vi "3_AdvancedDemo_TH260T3.vi"() -> ()   [LabVIEW 2017]
uses:
  Types/TH260_InputChannel.ctl
  Types/TH260_UIThread_Cmds.ctl
  Types/TH260_UIThread_Data.ctl
  _lib/PQ/TimeHarp260/TH260_InitInfo.ctl
  Types/TH260_DataProcThread_QData.ctl
  Types/TH260_DataProcThread_QCmds.ctl
  Types/TH260_VisThread_QData.ctl
  Types/TH260_VisThread_QCmds.ctl
  Types/TH260_VisThread_Data.ctl
  _lib/PQ/TimeHarp260/TH260_MeasMode.ctl
  _lib/PQ/TimeHarp260/TH260_TimingMode.ctl
  <vilib>/Utility/error.llb/DialogType.ctl
  _lib/PQ/TimeHarp260/th260lib_x86_x64_UIThread.llb/TH260_DllPath_global.vi
  <vilib>/Utility/error.llb/Error Cluster From Error Code.vi
  _lib/PQ/TimeHarp260/TH260_LibVersion_global.vi
  <vilib>/ErrorRing/Error Ring.xnode
panel:
  in  "Settings":bool=TRUE
  in  "Run continuously":bool caption="Conti."
  in  "Start":bool
  in  "Scale":bool
  out "CountRates":i32[](graph)
  in  "HistoAcqTime":dbl=1.0 caption="Int.Time    s" min=0.1 max=360000.0 step=0.1
  in  "AcqTime":i32=360000000 caption="T3Acq.   ms" min=1 max=360000 step=1
  in  "Binning":i32(ring) caption="Resol.      ps" items=["250", "500", "1000", "2000", "4000", "8000", "16000", "32000", "64000", "128000", "256000", "512000", "1024000", "2048000", "4096000", "8192000", "16384000", "32768000", "65536000", "131072000", "262144000", "524288000"]
  in  "HistoOffset":i32 caption="Offset      ns" min=0 max=500000 step=1
  out "DeltaT":dbl=inf caption="Resol.     ms" format="%.2f"
  in  "BitShift":i32=15 min=0 max=32 step=1
  in  "OvlLevel":u32=65536 caption="Ovl.Level" min=1024 max=65536 step=1024
  in  "StopOvl.":bool=TRUE
  out "TTraceGraph":T1(graph)
  out "HistoGraph":cluster{dbl, "Resol":dbl, "Histos":u32[][]}(graph)
  in  "SyncTrgEdge":i32(ring) caption="Edge" items=["falling", "rising"]
  in  "SyncTrgLevel":i32=-100 caption="Level        mV" min=-1200 max=1200 step=1
  in  "SyncCFDLevel":i32=-100 caption="Level        mV" min=-1200 max=0 step=1
  in  "SyncZeroX":i32=-10 caption="ZeroCr.    mV" min=-40 max=0 step=1
  in  "SyncDivider":i32(ring)=3 caption="Divider" items=["1", "2", "4", "8"]
  in  "SyncOffset":i32 caption="Offset        ps" min=-99999 max=99999 step=1
  in  "Channels":T2[](array[typedef])=[{"Name"="Inp.Chan 1", "Enable"=TRUE, "Offset"=0, "CFDLevel"=50, "ZeroX"=10, "dtcode"=0, "TrgLevel"=-100, "TrgEdge"=0}, {"Name"="Inp.Chan 2", "Enable"=TRUE, "Offset"=0, "CFDLevel"=50, "ZeroX"=10, "dtcode"=0, "TrgLevel"=-100, "TrgEdge"=0}, {"Name"="Inp.Chan 3", "Enable"=TRUE, "Offset"=0, "CFDLevel"=50, "ZeroX"=10, "dtcode"=0, "TrgLevel"=-100, "TrgEdge"=0}, {"Name"="Inp.Chan 4", "Enable"=TRUE, "Offset"=0, "CFDLevel"=50, "ZeroX"=10, "dtcode"=0, "TrgLevel"=-100, "TrgEdge"=0}, {"Name"="Inp.Chan 5", "Enable"=TRUE, "Offset"=0, "CFDLevel"=50, "ZeroX"=10, "dtcode"=0, "TrgLevel"=-100, "TrgEdge"=0}, {"Name"="Inp.Chan 6", "Enable"=TRUE, "Offset"=0, "CFDLevel"=50, "ZeroX"=10, "dtcode"=0, "TrgLevel"=-100, "TrgEdge"=0}, {"Name"="Inp.Chan 7", "Enable"=TRUE, "Offset"=0, "CFDLevel"=50, "ZeroX"=10, "dtcode"=0, "TrgLevel"=-100, "TrgEdge"=0}, {"Name"="Inp.Chan 8", "Enable"=TRUE, "Offset"=0, "CFDLevel"=50, "ZeroX"=10, "dtcode"=0, "TrgLevel"=-100, "TrgEdge"=0}] {"TrgEdge" items=["falling", "rising"]; "TrgLevel" min=-1200 max=1200 step=1; "dtcode" items=["24", "44", "66", "88", "112", "135", "160", "180"]; "ZeroX" min=-40 max=0 step=1; "Offset" min=-99999 max=99999 step=1; "CFDLevel" min=-1200 max=0 step=1}
  out "SyncRate":string="Sync Rate: 0 cps\n"
  out "OverRun":bool caption="Overrun:"
  out "Status":string="Elements in Q: 0"
  # "Histogram"
  # "Time Trace"
  # "Sync"
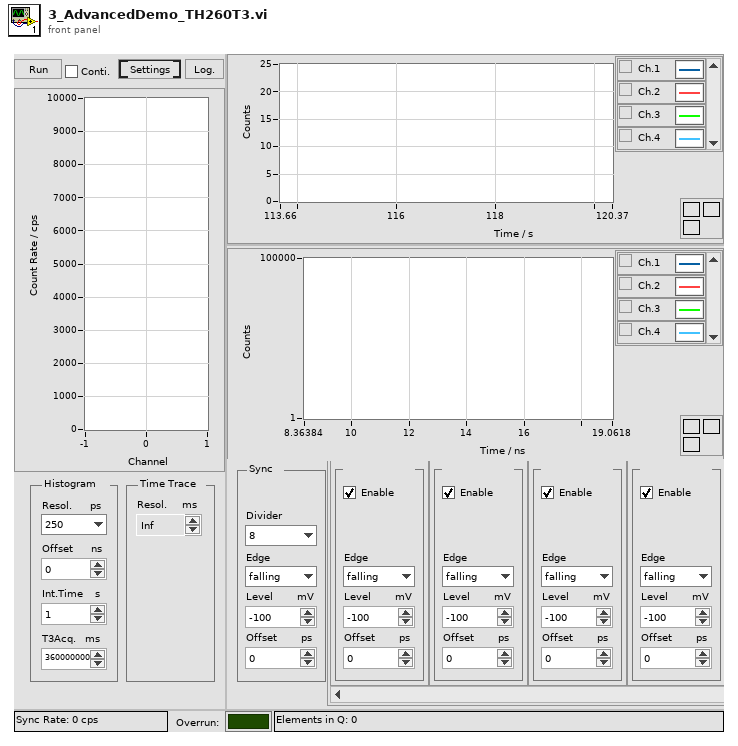
[diagram p1: front panel]
types:
  T1 = cluster{dbl, "Resolution":dbl, "Histogram":u32[][]}
  T2 = typedef "TH260_InputChannel.ctl" = cluster{"Name":string, "Enable":bool, "Offset":i32, "CFDLevel":i32, "ZeroX":i32, "dtcode":i32, "TrgLevel":i32, "TrgEdge":i32}
  T3 = typedef "TH260_DataProcThread_QCmds.ctl" = enum16{"Exit", "Proc", "Init", "SetShift", "SetNumChannels", "SetHistAcqTime"}
  T4 = typedef "TH260_VisThread_Data.ctl" = cluster{"Resol":dbl, "DeltaT":dbl, "NumChannels":i32}
  T5 = typedef "TH260_VisThread_QData.ctl" = cluster{"Histos":u32[][], "Cmd":T6, "TimeTrace":u32[][], "Bin":i32, "Total bin":u64, "Status":string, "Resol":dbl, "DeltaT":dbl, "nChannels":i32}
  T6 = typedef "TH260_VisThread_QCmds.ctl" = enum16{"_none_", "Resol", "nChannels", "DeltaT", "Histo", "TTrace", "Status"}
  T7 = typedef "TH260_DataProcThread_QData.ctl" = cluster{"Cmd":T3, "nActual":i32, "Buffer":u32[], "TickCount":u32, "Param":i32}
  T8 = typedef "TH260_UIThread_Data.ctl" = cluster{"Init Info":T9, "DevIdx":i32, "Channels":T2[], "CurrentChannels":i32[], "AcqTime":i32, "Binning":i32, "HistoOffset":i32, "HistoLen":i32, "StopOvl.":bool, "OvlLevel":u32, "StartMeas":bool, "HistoLength":i32, "Resolution":dbl, "Run cont.":bool, "Status":string, "SyncRate":i32, "BitShift":i32, "HistoAcqTime":dbl, "SyncTrgEdge":i32, "SyncTrgLevel":i32, "SyncCFDLevel":i32, "SyncZeroX":i32, "SyncDivider":i32, "SyncOffset":i32}
  T9 = typedef "TH260_InitInfo.ctl" = cluster{"Library Version":string, "Serial No.":string, "Model":string, "Partnum":string, "Version":string, "features":i32, "nchannels":i32, "Base Resolution":dbl, "Bin Steps":i32}
  T10 = typedef "TH260_UIThread_Cmds.ctl" = enum16{"Idle", "Init", "SetInpChanEnable", "SetInpChanOffset", "SetInpChanCFD", "SetInpChanTrg", "SetInpChanDeadtime", "SetSyncDivider", "SetSyncCFD", "SetSyncTrg", "SetSyncOffset", "SetBinning", "SetHistoOffset", "SetHistoLen", "SetStopOvl", "SetBitShift", "SetHistoAcqTime", "GetRates", "StartMeas", "StopMeas", "AbortMeas", "GetResolution", "GetHisto", "ReadFiFo", "WriteStatus", "Resize", "EnableControls", "DisableControls", "Error", "Exit"}
  T11 = enum8{"Enabled", "Disabled", "Disabled and Grayed Out"}
  T12 = typedef "TH260_TimingMode.ctl" = i32
  T13 = typedef "TH260_MeasMode.ctl" = i32
  T14 = typedef "DialogType.ctl" = u16
  T15 = cluster{"T0":dbl, "dt":dbl, "TimeTrace_out":u32[][]}
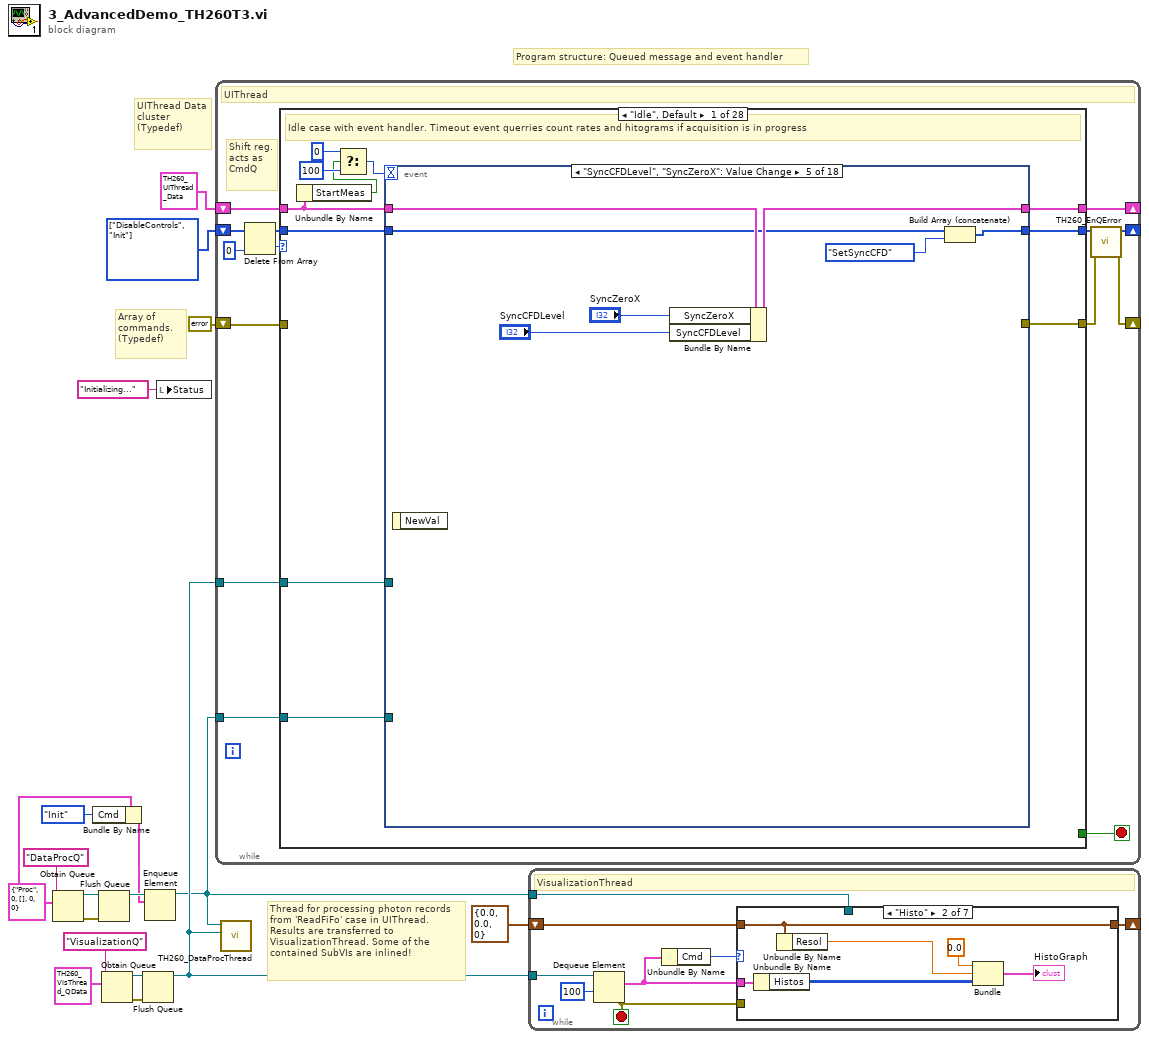
[diagram p0: block diagram]
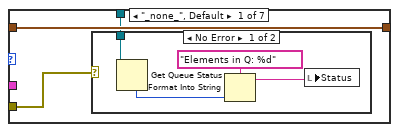
[diagram p2: hidden frame]
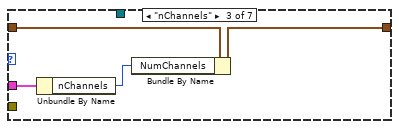
[diagram p4: hidden frame]
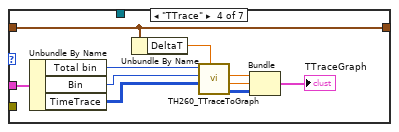
[diagram p5: hidden frame]
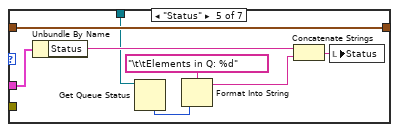
[diagram p6: hidden frame]
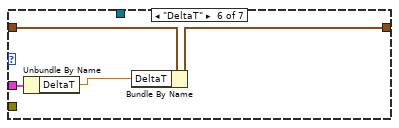
[diagram p7: hidden frame]
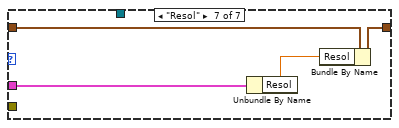
[diagram p8: hidden frame]
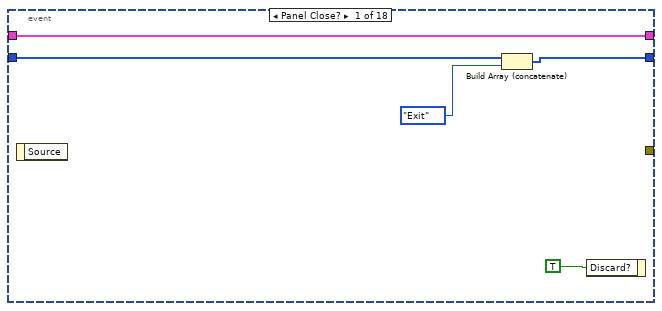
[diagram p9: hidden frame]
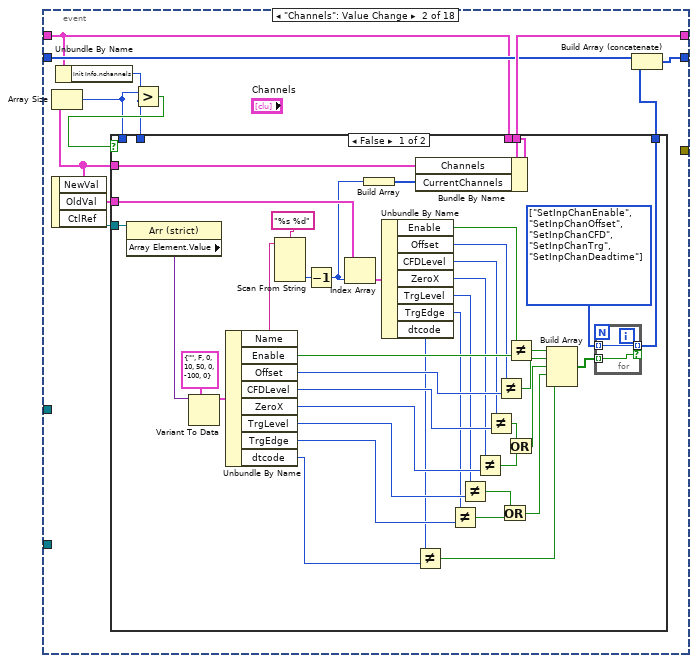
[diagram p10: hidden frame]
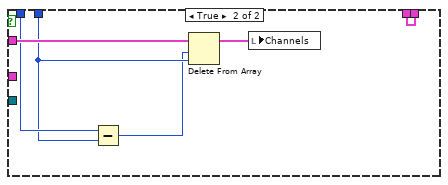
[diagram p11: hidden frame]
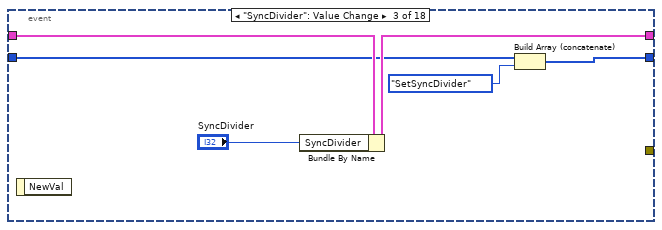
[diagram p12: hidden frame]
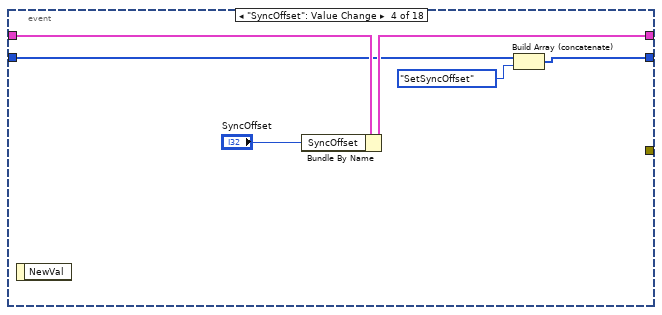
[diagram p13: hidden frame]
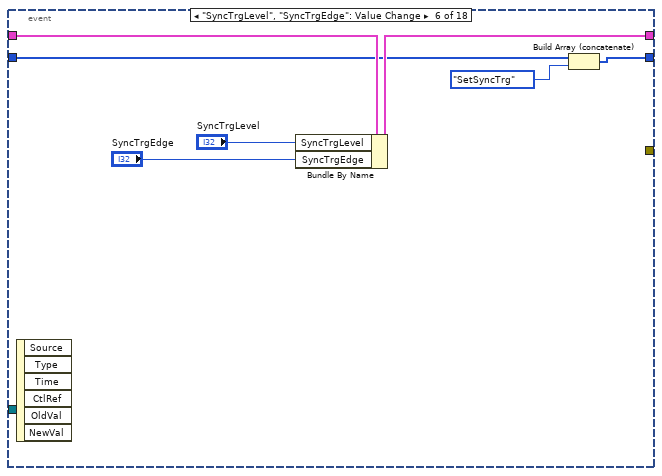
[diagram p14: hidden frame]
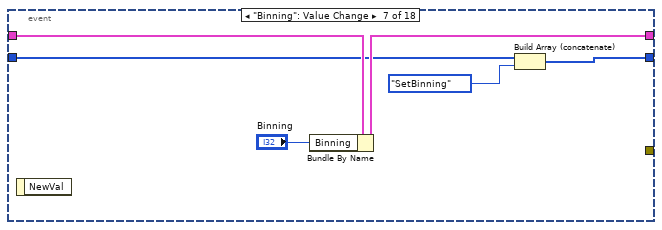
[diagram p15: hidden frame]
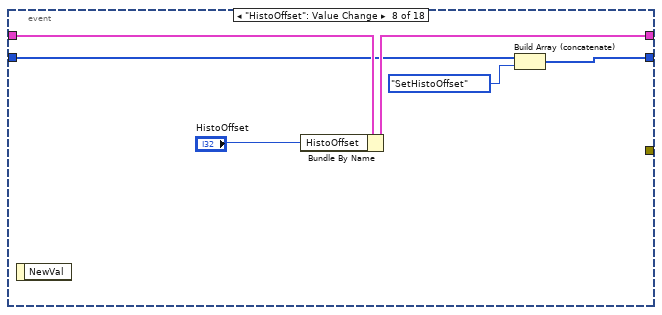
[diagram p16: hidden frame]
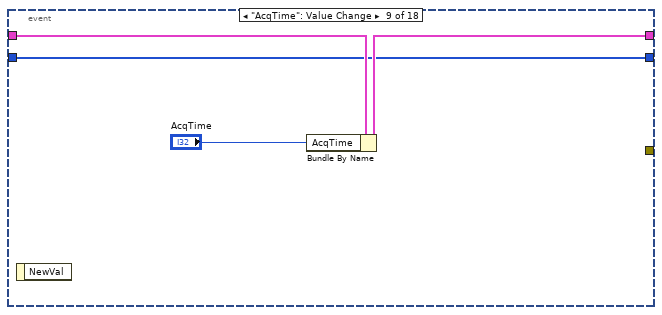
[diagram p17: hidden frame]
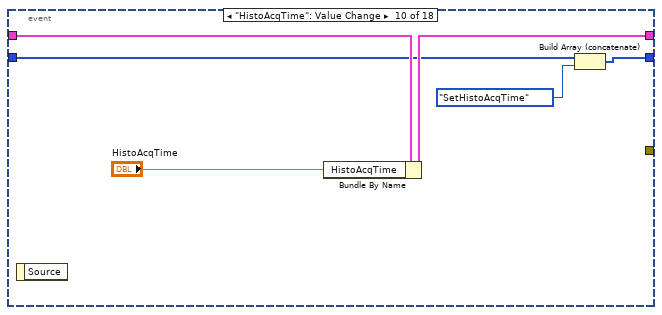
[diagram p18: hidden frame]
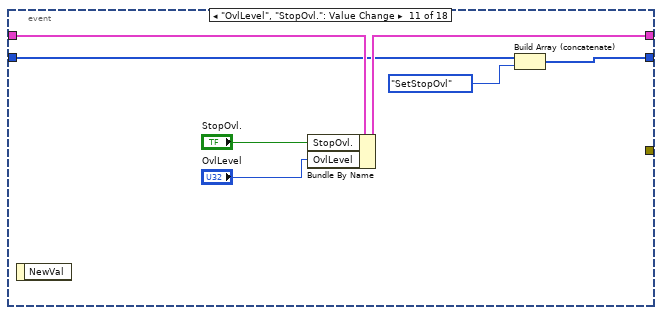
[diagram p19: hidden frame]
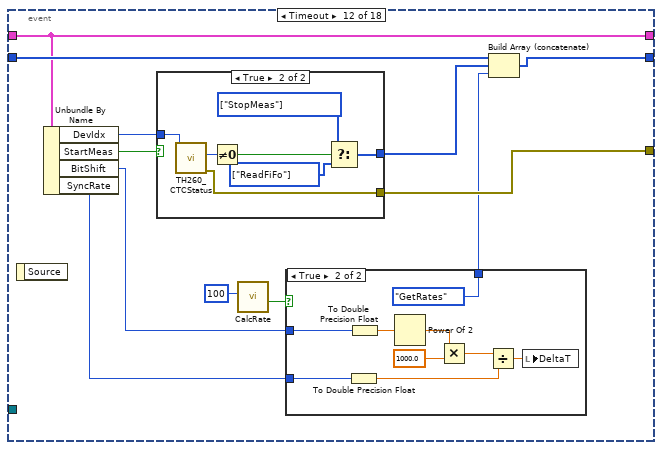
[diagram p20: hidden frame]
diagram:
  w4 = T7 {"Cmd"=enum."Proc", "nActual"=0, "Buffer"=[], "TickCount"=0, "Param"=0} ("MH_DataProcThread_QData")
  w17 = T10[] [enum."DisableControls", enum."Init"] items=["Idle", "Init", "SetInpChanEnable", "SetInpChanOffset", "SetInpChanCFD", "SetInpChanTrg", "SetInpChanDeadtime", "SetSyncDivider", "SetSyncCFD", "SetSyncTrg", "SetSyncOffset", "SetBinning", "SetHistoOffset", "SetHistoLen", "SetStopOvl", "SetBitShift", "SetHistoAcqTime", "GetRates", "StartMeas", "StopMeas", "AbortMeas", "GetResolution", "GetHisto", "ReadFiFo", "WriteStatus", "Resize", "EnableControls", "DisableControls", "Error", "Exit"]
  # "Thread for processing photon records from 'ReadFiFo' case in UIThread. Results are transferred to VisualizationThread. Some of the contained SubVIs are inlined!"
  # "Array of commands.\n(Typedef)"
  # "Program structure: Queued message and event handler"
  # "UIThread Data cluster\n(Typedef)"
  n1 = Obtain Queue(name (unnamed)="DataProcQ", element data type=w4) -> (queue out=w14:refnum<queue>, error out=w13:errorcluster)  [unwired: 3 in, 1 out]
  n2 = Bundle By Name(cluster=w4, "Cmd"=TH260_DataProcThread_QCmds."Init") -> (w2:T7)
  n3 = Flush Queue(queue=w14, error in (no error)=w13) -> (queue out=w5:refnum<queue>)  [unwired: 2 out]
  n4 = Obtain Queue(name (unnamed)="VisualizationQ", element data type=T5 {"Histos"=[], "Cmd"=enum."_none_", "TimeTrace"=[], "Bin"=0, "Total bin"=0, "Status"="", "Resol"=0.0, "DeltaT"=0.0, "nChannels"=0} ("MH_GUIThread_QData")) -> (queue out=w12:refnum<queue>, error out=w11:errorcluster)  [unwired: 3 in, 1 out]
  n5 = Flush Queue(queue=w12, error in (no error)=w11) -> (queue out=w7:refnum<queue>)  [unwired: 2 out]
  n6 = Enqueue Element(queue=w5, element=w2) -> (queue out=w1:refnum<queue>)  [unwired: 2 in, 2 out]
  n7 = local write "Status"("Initializing..." ("Status")) -> ()
  n8 = while {
    shift-right: [w21] -> _
    shift-left: w17 -> [w28]
    shift-right: [w31] -> _
    shift-left: T8 {"Init Info"={"Library Version"="", "Serial No."="", "Model"="", "Partnum"="", "Version"="", "features"=0, "nchannels"=0, "Base Resolution"=0.0, "Bin Steps"=0}, "DevIdx"=0, "Channels"=[], "CurrentChannels"=[], "AcqTime"=1, "Binning"=1, "HistoOffset"=1, "HistoLen"=1024, "StopOvl."=FALSE, "OvlLevel"=1024, "StartMeas"=FALSE, "HistoLength"=0, "Resolution"=0.0, "Run cont."=FALSE, "Status"="", "SyncRate"=0, "BitShift"=0, "HistoAcqTime"=0.0, "SyncTrgEdge"=50, "SyncTrgLevel"=0, "SyncCFDLevel"=-100, "SyncZeroX"=10, "SyncDivider"=1, "SyncOffset"=0} -> [w30]
    shift-right: [w23] -> _
    shift-left: errorcluster {"status"=FALSE, "code"=0, "source"=""} ("error IO") -> [w29]
    tunnel: w1 -> [w20]
    tunnel: w7 -> [w19]
    stop <- w32 stop-if-true
    # "Shift reg.\nacts as\nCmdQ"
    # "UIThread"
    n9 = Delete From Array(array=w28, index=0) -> (deleted portion=w26:T10, array with subset deleted=w25:T10[])  [unwired: 1 in]
    n10 = case shown="\"Idle\", Default" w26 {
      tunnel: [w43 w297 w331 w345 w359 w374 w389 w405 w414 w420 w422 w429 w437 w443 w463 w475 w487 w507 w513 w526 w543 w544 w570 w583 w590 w602 w608 w614] -> w22
      tunnel: [_ _ _ _ _ _ _ _ _ _ _ _ _ _ _ _ _ _ _ _ _ _ _ _ _ _ _ TRUE] -> w32
      tunnel: [w42 w278 w334 w348 w362 w377 w392 w407 w415 w421 w426 w433 w438 w444 w448 w465 w477 w511 w516 w528 w539 w554 w569 w571 w589 w601 w609 w617] -> w31
      tunnel: w30 -> [w39 w283 w334 w348 w362 w377 w392 w407 w415 w421 w426 w433 w438 w444 w448 w465 w478 w511 w517 w529 w540 w554 w569 w571 w589 w601 w609 w617]
      tunnel: [w40 w301 w332 w346 w360 w375 w390 w403 w413 w419 w425 w432 w436 w442 _ _ w486 w510 w519 w531 w541 w549 _ _ _ _ _ w615] -> w24
      tunnel: w29 -> [_ _ _ _ _ _ _ _ _ _ _ _ _ _ _ _ _ _ _ _ _ _ _ _ _ _ w610 _]
      tunnel: w25 -> [w41 w298 w331 w345 w359 w374 w389 w405 w414 w420 w422 w428 w437 w443 w463 w475 w487 w508 w514 w526 w543 w545 w570 w583 w590 w602 _ w614]
      tunnel: w20 -> [w34 w276 _ _ _ _ _ _ _ _ _ _ _ _ w449 w466 _ w504 _ _ _ w546 _ _ _ _ _ w613]
      tunnel: w19 -> [w33 w268 _ _ _ _ _ _ _ _ _ _ _ _ w450 _ _ _ _ _ w536 _ _ _ _ _ _ w612]
      frame "Idle", Default {
        # "Idle case with event handler. Timeout event querries count rates and hitograms if acquisition is in progress"
        n11 = Unbundle By Name(w39) -> ("StartMeas"=w37:bool)
        n12 = Select(t=0, s=w37, f=100) -> (s? t:f=w36:i32)
        n13 = event shown="[4] \"SyncCFDLevel\", \"SyncZeroX\": Value Change" {
          selector: _ -> [_ _ _ _ _ _ _ _ _ _ _ _ _ _ _ _ _ _]
          dyn-events: _ -> [_ _ _ _ _ _ _ _ _ _ _ _ _ _ _ _ _ _]
          timeout: w36 -> [_ _ _ _ _ _ _ _ _ _ _ _ _ _ _ _ _ _]
          tunnel: [w44 w54 w109 w115 w122 w129 w135 w141 w146 w151 w158 w173 w191 w203 w221 w227 w235 w245] -> w43
          tunnel: [w47 w57 w112 w118 w125 w132 w138 w144 w148 w154 w161 w172 w195 w202 w219 w226 w234 w248] -> w42
          tunnel: w39 -> [w47 w53 w113 w119 w126 w133 w139 w145 w149 w155 w162 w172 w196 w200 w220 w226 w234 w248]
          tunnel: w41 -> [w46 w56 w111 w117 w124 w131 w137 w143 w146 w152 w160 w174 w192 w204 w221 w227 w235 w246]
          tunnel: [_ _ _ _ _ _ _ _ _ _ _ w168 _ _ _ _ _ _] -> w40
          tunnel: w34 -> [_ _ _ _ _ _ _ _ _ _ _ _ _ _ _ _ _ _]
          tunnel: w33 -> [_ _ _ _ _ _ _ _ _ _ _ _ _ _ _ _ _ _]
          event Panel Close? {
            n14 = event-data() -> ()  [unwired: 1 in, 1 out]
            n15 = Build Array (concatenate)(w46, TH260_UIThread_Cmds."Exit") -> (w44:T10[])
            n16 = event-data("Discard?"=TRUE) -> ()  [unwired: 1 in, 1 out]
          }
          event "Channels": Value Change {
            n17 = event-data() -> ("NewVal"=w52:T2[], "OldVal"=w58:T2[], "CtlRef"=w59:refnum<vi>)  [unwired: 1 in]
            n18 = Array Size(array=w52) -> (size(s)=w49:i32)
            n19 = Unbundle By Name(w53) -> ("Init Info.nchannels"=w50:i32)
            n20 = Greater?(x=w49, y=w50) -> (0:w51:bool)
            n21 = case shown="False" w51 {
              tunnel: w59 -> [w99 _]
              tunnel: w58 -> [w93 _]
              tunnel: [w76 w107] -> w57
              tunnel: [w74 _] -> w55
              tunnel: w53 -> [w71 w107]
              tunnel: w52 -> [w70 w106]
              tunnel: w50 -> [_ w104]
              tunnel: w49 -> [_ w105]
              frame False {
                w77 = T10[] [enum."SetInpChanEnable", enum."SetInpChanOffset", enum."SetInpChanCFD", enum."SetInpChanTrg", enum."SetInpChanDeadtime"] items=["Idle", "Init", "SetInpChanEnable", "SetInpChanOffset", "SetInpChanCFD", "SetInpChanTrg", "SetInpChanDeadtime", "SetSyncDivider", "SetSyncCFD", "SetSyncTrg", "SetSyncOffset", "SetBinning", "SetHistoOffset", "SetHistoLen", "SetStopOvl", "SetBitShift", "SetHistoAcqTime", "GetRates", "StartMeas", "StopMeas", "AbortMeas", "GetResolution", "GetHisto", "ReadFiFo", "WriteStatus", "Resize", "EnableControls", "DisableControls", "Error", "Exit"]
                n22 = property class="Arr (strict)"(reference=w99) -> ("Array Element.Value"=w98:variant)  [unwired: 1 in, 2 out]
                n23 = Variant To Data(type=T2 {"Name"="", "Enable"=FALSE, "Offset"=0, "CFDLevel"=10, "ZeroX"=50, "dtcode"=0, "TrgLevel"=-100, "TrgEdge"=0} ("Channel"), Variant=w98) -> (data=w75:T2)  [unwired: 1 in, 1 out]
                n24 = Unbundle By Name(w75) -> ("Name"=w96:string, "Enable"=w90:bool, "Offset"=w88:i32, "CFDLevel"=w86:i32, "ZeroX"=w84:i32, "TrgLevel"=w68:i32, "TrgEdge"=w66:i32, "dtcode"=w61:i32)
                n25 = Scan From String(format string="%s %d", input string=w96) -> (output 2=w94:i32)  [unwired: 5 in, 3 out]
                n26 = Decrement(x=w94) -> (x-1=w73:i32)
                n27 = Index Array(array=w93, index=w73) -> (element=w92:T2)
                n28 = Build Array(w73) -> (w72:i32[])
                n29 = Unbundle By Name(w92) -> ("Enable"=w91:bool, "Offset"=w89:i32, "CFDLevel"=w87:i32, "ZeroX"=w85:i32, "TrgLevel"=w69:i32, "TrgEdge"=w67:i32, "dtcode"=w62:i32)
                n30 = Not Equal?(x=w62, y=w61) -> (x != y?=w60:bool)
                n31 = Bundle By Name(cluster=w71, "Channels"=w70, "CurrentChannels"=w72) -> (w76:T8)
                n32 = Not Equal?(x=w67, y=w66) -> (x != y?=w64:bool)
                n33 = Not Equal?(x=w69, y=w68) -> (x != y?=w65:bool)
                n34 = Not Equal?(x=w85, y=w84) -> (x != y?=w79:bool)
                n35 = Not Equal?(x=w87, y=w86) -> (x != y?=w80:bool)
                n36 = Not Equal?(x=w89, y=w88) -> (x != y?=w82:bool)
                n37 = Or(x=w65, y=w64) -> (x .or. y?=w63:bool)
                n38 = Not Equal?(x=w91, y=w90) -> (x != y?=w83:bool)
                n39 = Or(x=w80, y=w79) -> (x .or. y?=w78:bool)
                n40 = Build Array(w83, w82, w78, w63, w60) -> (w81:bool[])
                n41 = for {
                  tunnel: w81 -> [w100] mode=indexing
                  tunnel: w77 -> [w101] mode=indexing
                  tunnel: [w101] -> w74 mode=indexing if=w100
                }
              }
              frame True {
                n42 = Subtract(x=w105, y=w104) -> (x-y=w103:i32)
                n43 = Delete From Array(array=w106, length=w103, index=w104) -> (array with subset deleted=w102:T2[])  [unwired: 1 out]
                n44 = local write "Channels"(w102) -> ()
              }
            }
            n45 = Build Array (concatenate)(w56, w55) -> (w54:T10[])
          }
          event "SyncDivider": Value Change {
            n46 = event-data() -> ()  [unwired: 1 in, 1 out]
            n47 = Bundle By Name(cluster=w113, "SyncDivider"="SyncDivider") -> (w112:T8)
            n48 = Build Array (concatenate)(w111, TH260_UIThread_Cmds."SetSyncDivider") -> (w109:T10[])
          }
          event "SyncOffset": Value Change {
            n49 = event-data() -> ()  [unwired: 1 in, 1 out]
            n50 = Bundle By Name(cluster=w119, "SyncOffset"="SyncOffset") -> (w118:T8)
            n51 = Build Array (concatenate)(w117, TH260_UIThread_Cmds."SetSyncOffset") -> (w115:T10[])
          }
          event "SyncCFDLevel", "SyncZeroX": Value Change {
            n52 = event-data() -> ()  [unwired: 1 in, 1 out]
            n53 = Bundle By Name(cluster=w126, "SyncZeroX"="SyncZeroX", "SyncCFDLevel"="SyncCFDLevel") -> (w125:T8)
            n54 = Build Array (concatenate)(w124, TH260_UIThread_Cmds."SetSyncCFD") -> (w122:T10[])
          }
          event "SyncTrgLevel", "SyncTrgEdge": Value Change {
            n55 = event-data() -> ()  [unwired: 1 in, 6 out]
            n56 = Bundle By Name(cluster=w133, "SyncTrgLevel"="SyncTrgLevel", "SyncTrgEdge"="SyncTrgEdge") -> (w132:T8)
            n57 = Build Array (concatenate)(w131, TH260_UIThread_Cmds."SetSyncTrg") -> (w129:T10[])
          }
          event "Binning": Value Change {
            n58 = event-data() -> ()  [unwired: 1 in, 1 out]
            n59 = Bundle By Name(cluster=w139, "Binning"="Binning") -> (w138:T8)
            n60 = Build Array (concatenate)(w137, TH260_UIThread_Cmds."SetBinning") -> (w135:T10[])
          }
          event "HistoOffset": Value Change {
            n61 = event-data() -> ()  [unwired: 1 in, 1 out]
            n62 = Bundle By Name(cluster=w145, "HistoOffset"="HistoOffset") -> (w144:T8)
            n63 = Build Array (concatenate)(w143, TH260_UIThread_Cmds."SetHistoOffset") -> (w141:T10[])
          }
          event "AcqTime": Value Change {
            n64 = event-data() -> ()  [unwired: 1 in, 1 out]
            n65 = Bundle By Name(cluster=w149, "AcqTime"="AcqTime") -> (w148:T8)
          }
          event "HistoAcqTime": Value Change {
            n66 = event-data() -> ()  [unwired: 1 in, 1 out]
            n67 = Bundle By Name(cluster=w155, "HistoAcqTime"="HistoAcqTime") -> (w154:T8)
            n68 = Build Array (concatenate)(w152, TH260_UIThread_Cmds."SetHistoAcqTime") -> (w151:T10[])
          }
          event "OvlLevel", "StopOvl.": Value Change {
            n69 = event-data() -> ()  [unwired: 1 in, 1 out]
            n70 = Bundle By Name(cluster=w162, "StopOvl."="StopOvl.", "OvlLevel"="OvlLevel") -> (w161:T8)
            n71 = Build Array (concatenate)(w160, TH260_UIThread_Cmds."SetStopOvl") -> (w158:T10[])
          }
          event Timeout {
            n72 = event-data() -> ()  [unwired: 1 in, 1 out]
            n73 = Unbundle By Name(w172) -> ("DevIdx"=w170:i32, "StartMeas"=w171:bool, "BitShift"=w167:i32, "SyncRate"=w166:i32)
            n74 = case shown="True" w171 {
              tunnel: w170 -> [_ w190]
              tunnel: [_ w188] -> w169
              tunnel: [_ w185] -> w168
              frame False {
              }
              frame True {
                w186 = T10[] [enum."ReadFiFo"] items=["Idle", "Init", "SetInpChanEnable", "SetInpChanOffset", "SetInpChanCFD", "SetInpChanTrg", "SetInpChanDeadtime", "SetSyncDivider", "SetSyncCFD", "SetSyncTrg", "SetSyncOffset", "SetBinning", "SetHistoOffset", "SetHistoLen", "SetStopOvl", "SetBitShift", "SetHistoAcqTime", "GetRates", "StartMeas", "StopMeas", "AbortMeas", "GetResolution", "GetHisto", "ReadFiFo", "WriteStatus", "Resize", "EnableControls", "DisableControls", "Error", "Exit"]
                w187 = T10[] [enum."StopMeas"] items=["Idle", "Init", "SetInpChanEnable", "SetInpChanOffset", "SetInpChanCFD", "SetInpChanTrg", "SetInpChanDeadtime", "SetSyncDivider", "SetSyncCFD", "SetSyncTrg", "SetSyncOffset", "SetBinning", "SetHistoOffset", "SetHistoLen", "SetStopOvl", "SetBitShift", "SetHistoAcqTime", "GetRates", "StartMeas", "StopMeas", "AbortMeas", "GetResolution", "GetHisto", "ReadFiFo", "WriteStatus", "Resize", "EnableControls", "DisableControls", "Error", "Exit"]
                n75 = call "TH260_CTCStatus.vi"("devidx"=w190) -> ("error out"=w185:errorcluster, "ctcstatus"=w189:i32)  [unwired: 8 in, 1 out]
                n76 = Not Equal To 0?(x=w189) -> (x != 0?=w184:bool)
                n77 = Select(t=w187, s=w184, f=w186) -> (s? t:f=w188:T10[])
              }
            }
            n78 = call "CalcRate.vi"("Refresh(ms)"=u32 100) -> ("updated?"=w164:bool)  [unwired: 8 in, 2 out]
            n79 = case shown="True" w164 {
              tunnel: w167 -> [_ w177]
              tunnel: w166 -> [_ w176]
              tunnel: [_ TH260_UIThread_Cmds."GetRates"] -> w165
              frame False {
              }
              frame True {
                n80 = To Double Precision Float(number=w176) -> (double precision float=w181:dbl)
                n81 = To Double Precision Float(number=w177) -> (double precision float=w182:dbl)
                n82 = Power Of 2(x=w182) -> (2^x=w180:dbl)
                n83 = Multiply(x=w180, y=1000.0) -> (x*y=w179:dbl)
                n84 = Divide(x=w179, y=w181) -> (x/y=w183:dbl)
                n85 = local write "DeltaT"(w183) -> ()
              }
            }
            n86 = Build Array (concatenate)(w174, w169, w165) -> (w173:T10[])
          }
          event "BitShift": Value Change {
            n87 = event-data() -> ()  [unwired: 1 in, 1 out]
            n88 = Bundle By Name(cluster=w196, "BitShift"="BitShift") -> (w195:T8)
            n89 = Build Array (concatenate)(w192, TH260_UIThread_Cmds."SetBitShift") -> (w191:T10[])
          }
          event "Start": Value Change {
            n90 = event-data() -> ()  [unwired: 1 in, 1 out]
            n91 = Unbundle By Name(w200) -> ("SyncRate"=w199:i32)
            n92 = Greater Or Equal?(x=w199, y=10) -> (x >= y?=w197:bool)
            n93 = case shown="True" w197 {
              selector: w197 -> [w206 _]
              tunnel: w204 -> [w208 w217]
              tunnel: [w208 w215] -> w203
              tunnel: [w207 w214] -> w202
              tunnel: "Start" -> [_ w213]
              tunnel: w200 -> [w207 w209]
              frame False {
                n94 = local write "Start"(w206) -> ()
                n95 = One Button Dialog(message="SyncRate too low!!!" ("Status")) -> ()  [unwired: 1 in, 1 out]
              }
              frame True {
                w212 = T10[] [enum."SetBitShift", enum."SetHistoAcqTime", enum."StartMeas"] items=["Idle", "Init", "SetInpChanEnable", "SetInpChanOffset", "SetInpChanCFD", "SetInpChanTrg", "SetInpChanDeadtime", "SetSyncDivider", "SetSyncCFD", "SetSyncTrg", "SetSyncOffset", "SetBinning", "SetHistoOffset", "SetHistoLen", "SetStopOvl", "SetBitShift", "SetHistoAcqTime", "GetRates", "StartMeas", "StopMeas", "AbortMeas", "GetResolution", "GetHisto", "ReadFiFo", "WriteStatus", "Resize", "EnableControls", "DisableControls", "Error", "Exit"]
                n96 = Bundle By Name(cluster=w209, "StartMeas"=w213) -> (w214:T8)
                n97 = Build Array(TH260_UIThread_Cmds."AbortMeas") -> (w210:T10[])
                n98 = Select(t=w212, s=w213, f=w210) -> (s? t:f=w216:T10[])
                n99 = Build Array (concatenate)(w217, w216) -> (w215:T10[])
              }
            }
          }
          event "Run continuously": Value Change {
            n100 = event-data() -> ()  [unwired: 1 in, 1 out]
            n101 = Bundle By Name(cluster=w220, "Run cont."="Run continuously") -> (w219:T8)
          }
          event "Scale": Value Change {
            n102 = event-data() -> ()  [unwired: 1 in, 1 out]
            n103 = Select(t=u8 0 ("Y Scale.Mapping Mode"), s="Scale", f=u8 1 ("Y Scale.Mapping Mode")) -> (s? t:f=w222:u8)
            n104 = property on="HistoGraph" class="WFGraph (strict)"("YScale.Mapping Mode"=w222) -> ()  [unwired: 2 in, 2 out]
          }
          event "Settings": Value Change {
            n105 = event-data() -> ()  [unwired: 1 in, 1 out]
            n106 = property on="Splitter" class="Splitter"() -> ("Position"=w233:i32)  [unwired: 2 in, 2 out]
            n107 = Select(t=250 ("PosT"), s="Settings", f=0 ("PosF")) -> (s? t:f=w230:i32)
            n108 = Subtract(x=w233, y=w230) -> (x-y=w229:i32)
            n109 = while {
              shift-right: [w244] -> _
              shift-left: w229 -> [w237]
              i -> [w243]
              stop <- w240 stop-if-true
              n110 = property on="Splitter 4" class="Splitter"("Position"=w237) -> (error out=w236:errorcluster)  [unwired: 2 in, 1 out]
              n111 = Greater Or Equal?(x=w243, y=10) -> (x >= y?=w241:bool)
              n112 = Decrement(x=w237) -> (x-1=w244:i32)
              n113 = Unbundle(w236) -> ("status"=w239:bool)  [unwired: 2 out]
              n114 = Not(x=w239) -> (.not. x?=w238:bool)
              n115 = Or(x=w238, y=w241) -> (x .or. y?=w240:bool)
            }
          }
          event Panel Resize {
            n116 = event-data() -> ()  [unwired: 1 in, 1 out]
            n117 = Build Array (concatenate)(w246, TH260_UIThread_Cmds."Resize") -> (w245:T10[])
          }
        }
      }
      frame "Init" {
        w254 = -100 ("SyncTrgLevel")
        w255 = 0 ("SyncTrgEdge")
        w257 = T12 0 items=["Hires", "Lowres"]  # TimingMode
        w258 = T13 3 items=["Histo"=0, "T2"=2, "T3"=3]  # MeasMode
        w266 = 1.0 ("HistoAcqTime")
        w267 = 15 ("Value (Signaling)")
        w285 = FALSE ("Run cont.")
        w287 = FALSE ("StartMeas")
        w288 = u32 100000 ("OvlLevel")
        w289 = TRUE ("StopOvl.")
        w290 = 360000000 ("AcqTime")
        w291 = 0 ("HistoOffset")
        w292 = 0 ("Binning")
        w293 = -100 ("SyncLevel")
        w294 = -10 ("SyncZeroX")
        w295 = 0 ("SyncOffset")
        w296 = 3 ("SyncDivider")
        # "100 x 60 x 60 x 1000 = 100 h"
        # "Init all FP controls and corresponding copy in UIThread Data cluster"
        # "EnQ list of commands"
        # "Array with Inp.Chan."
        # "Initialization: 1. Init HW -> get # of channels -> make array for Inp.Channels\n2. Init all FP controls and corresponding fields in UIThread Data cluster\n3. EnQ list of commands for further initialization"
        n118 = xnode "Error Ring"() -> ("error out"=w260:errorcluster)
        n119 = call "GetDLLPath.vi"("DllName_32bit"="TH260Lib.dll" ("name or relative path"), "DllName_64bit"="TH260Lib64.dll" ("name or relative path")) -> ("file exists?"=w262:bool, "DLLPath"=w263:path)  [unwired: 8 in]
        n120 = global write "TH260_DllPath_global.vi" "DllPath"(w263) -> ()
        n121 = Select(t=errorcluster {"status"=FALSE, "code"=0, "source"=""} ("error IO"), s=w262, f=w260) -> (s? t:f=w279:errorcluster)
        n122 = global read "TH260_LibVersion_global.vi" "Library Version"() -> (w259:string)
        n123 = property on="Settings" class="Bool (strict)"("Val(Sgnl)"=TRUE ("Value (Signaling)")) -> ()  [unwired: 2 in, 2 out]
        n124 = property on="Scale" class="Bool (strict)"("Val(Sgnl)"=FALSE ("Value (Signaling)")) -> ()  [unwired: 2 in, 2 out]
        n125 = call "InitTH260_UIThread.vi"("error in (no error)"=w279, "MeasMode"=w258, "TimingMode"=w257, "Library Version"=w259) -> ("error out"=w301:errorcluster, "Init Info"=w253:T9, "DevIdx"=w303:i32)  [unwired: 5 in]
        n126 = Unbundle By Name(w253) -> ("Model"=w252:string)
        n127 = local write "SyncDivider"(w296) -> ()
        n128 = local write "SyncOffset"(w295) -> ()
        n129 = local write "SyncZeroX"(w294) -> ()
        n130 = local write "SyncCFDLevel"(w293) -> ()
        n131 = local write "SyncTrgEdge"(w255) -> ()
        n132 = local write "SyncTrgLevel"(w254) -> ()
        n133 = Bundle By Name(cluster=w283, "DevIdx"=w303, "Status"="Initialized!", "Init Info"=w253) -> (w282:T8)
        n134 = Unbundle By Name(w282) -> ("Init Info.Bin Steps"=w281:i32, "Init Info.Base Resolution"=w256:dbl, "Init Info.nchannels"=w269:i32)
        n135 = for {
          N: w269 -> [_]
          tunnel: T2 {"Name"="", "Enable"=FALSE, "Offset"=0, "CFDLevel"=10, "ZeroX"=50, "dtcode"=0, "TrgLevel"=-100, "TrgEdge"=0} ("Channel") -> [w327]
          tunnel: [w326] -> w300 mode=indexing
          tunnel: [w316] -> w299 mode=indexing
          i -> [w316]
          # "Init values for Inp. Channels"
          n136 = Increment(x=w316) -> (x+1=w319:i32)
          n137 = Format Into String(format string="Ch.%d", w319) -> (resulting string=w317:string)  [unwired: 2 in, 1 out]
          n138 = Format Into String(format string="Inp.Chan %d", w319) -> (resulting string=w324:string)  [unwired: 2 in, 1 out]
          n139 = property on="HistoGraph" class="WFGraph (strict)"("Active Plot"=w316, "Plot.Plot Name"=w317) -> ()  [unwired: 2 in, 2 out]
          n140 = Bundle By Name(cluster=w327, "Name"=w324, "Enable"=TRUE, "Offset"=0, "CFDLevel"=-100 ("CFDZeroX"), "ZeroX"=-10 ("CFDLevel"), "dtcode"=0, "TrgLevel"=-100, "TrgEdge"=0) -> (w326:T2)
          n141 = property on="TTraceGraph" class="WFGraph (strict)"("Active Plot"=w316, "Plot.Plot Name"=w317) -> ()  [unwired: 2 in, 2 out]
        }
        n142 = Bundle By Name(cluster=T5 {"Histos"=[], "Cmd"=enum."_none_", "TimeTrace"=[], "Bin"=0, "Total bin"=0, "Status"="", "Resol"=0.0, "DeltaT"=0.0, "nChannels"=0} ("MH_GUIThread_QData"), "Cmd"=TH260_VisThread_QCmds."nChannels", "nChannels"=w269) -> (w271:T5)
        n143 = call "TH260_CalcBinningValues.vi"("BaseRes"=w256, "Bin Steps"=w281) -> ("BinningValues"=w286:cluster{"String":string, "Value":i32}[])  [unwired: 9 in]
        n144 = property on="Binning" class="Ring (strict)"("StringsAndValues[]"=w286) -> ()  [unwired: 2 in, 2 out]
        n145 = Bundle By Name(cluster=T7 {"Cmd"=enum."Proc", "nActual"=0, "Buffer"=[], "TickCount"=0, "Param"=0} ("MH_DataProcThread_QData"), "Param"=w269, "Cmd"=TH260_DataProcThread_QCmds."SetNumChannels") -> (w275:T7)
        n146 = Enqueue Element(queue=w268, element=w271) -> ()  [unwired: 2 in, 3 out]
        n147 = Enqueue Element(queue=w276, element=w275) -> ()  [unwired: 2 in, 3 out]
        n148 = local write "Channels"(w300) -> ()
        n149 = Bundle By Name(cluster=w282, "Channels"=w300, "CurrentChannels"=w299, "SyncDivider"=w296, "SyncOffset"=w295, "SyncZeroX"=w294, "SyncCFDLevel"=w293, "SyncTrgEdge"=w255, "SyncTrgLevel"=w254, "Binning"=w292, "HistoOffset"=w291, "AcqTime"=w290, "StopOvl."=w289, "OvlLevel"=w288, "StartMeas"=w287, "Run cont."=w285, "BitShift"=w267, "HistoAcqTime"=w266) -> (w278:T8)
        n150 = case shown="\"TimeHarp 260 P\"" w252 {
          tunnel: [FALSE TRUE] -> w251
          tunnel: [w304 w306] -> w249
          frame Default {
            w304 = T10[] [enum."SetSyncDivider", enum."SetSyncOffset", enum."SetSyncTrg", enum."SetInpChanEnable", enum."SetInpChanOffset", enum."SetInpChanTrg", enum."SetBinning", enum."SetHistoOffset", enum."Resize", enum."EnableControls", enum."GetRates", enum."SetBitShift", enum."SetHistoAcqTime", enum."WriteStatus"] items=["Idle", "Init", "SetInpChanEnable", "SetInpChanOffset", "SetInpChanCFD", "SetInpChanTrg", "SetInpChanDeadtime", "SetSyncDivider", "SetSyncCFD", "SetSyncTrg", "SetSyncOffset", "SetBinning", "SetHistoOffset", "SetHistoLen", "SetStopOvl", "SetBitShift", "SetHistoAcqTime", "GetRates", "StartMeas", "StopMeas", "AbortMeas", "GetResolution", "GetHisto", "ReadFiFo", "WriteStatus", "Resize", "EnableControls", "DisableControls", "Error", "Exit"]
          }
          frame "TimeHarp 260 P" {
            w306 = T10[] [enum."SetSyncDivider", enum."SetSyncOffset", enum."SetSyncCFD", enum."SetInpChanEnable", enum."SetInpChanOffset", enum."SetInpChanCFD", enum."SetInpChanDeadtime", enum."SetBinning", enum."SetHistoOffset", enum."Resize", enum."EnableControls", enum."GetRates", enum."SetBitShift", enum."SetHistoAcqTime", enum."WriteStatus"] items=["Idle", "Init", "SetInpChanEnable", "SetInpChanOffset", "SetInpChanCFD", "SetInpChanTrg", "SetInpChanDeadtime", "SetSyncDivider", "SetSyncCFD", "SetSyncTrg", "SetSyncOffset", "SetBinning", "SetHistoOffset", "SetHistoLen", "SetStopOvl", "SetBitShift", "SetHistoAcqTime", "GetRates", "StartMeas", "StopMeas", "AbortMeas", "GetResolution", "GetHisto", "ReadFiFo", "WriteStatus", "Resize", "EnableControls", "DisableControls", "Error", "Exit"]
          }
        }
        n151 = Not(x=w251) -> (.not. x?=w250:bool)
        n152 = property on="dtcode" class="Ring (strict)"("Visible"=w251) -> ()  [unwired: 2 in, 2 out]
        n153 = property on="SyncZeroX" class="DigNum (strict)"("Visible"=w251) -> ()  [unwired: 2 in, 2 out]
        n154 = property on="SyncCFDLevel" class="DigNum (strict)"("Visible"=w251) -> ()  [unwired: 2 in, 2 out]
        n155 = local write "Binning"(w292) -> ()
        n156 = local write "HistoOffset"(w291) -> ()
        n157 = local write "StopOvl."(w289) -> ()
        n158 = local write "OvlLevel"(w288) -> ()
        n159 = local write "Start"(w287) -> ()
        n160 = local write "Run continuously"(w285) -> ()
        n161 = local write "BitShift"(w267) -> ()
        n162 = local write "AcqTime"(w290) -> ()
        n163 = local write "HistoAcqTime"(w266) -> ()
        n164 = property on="CFDLevel" class="DigNum (strict)"("Visible"=w251) -> ()  [unwired: 2 in, 2 out]
        n165 = property on="ZeroX" class="DigNum (strict)"("Visible"=w251) -> ()  [unwired: 2 in, 2 out]
        n166 = property on="SyncTrgLevel" class="DigNum (strict)"("Visible"=w250) -> ()  [unwired: 2 in, 2 out]
        n167 = property on="SyncTrgEdge" class="Ring (strict)"("Visible"=w250) -> ()  [unwired: 2 in, 2 out]
        n168 = property on="TrgLevel" class="DigNum (strict)"("Visible"=w250) -> ()  [unwired: 2 in, 2 out]
        n169 = property on="TrgEdge" class="Ring (strict)"("Visible"=w250) -> ()  [unwired: 2 in, 2 out]
        n170 = Build Array (concatenate)(w298, w249) -> (w297:T10[])
      }
      frame "SetInpChanEnable" {
        n171 = Unbundle By Name(w334) -> ("DevIdx"=w333:i32, "Channels"=w328:T2[], "CurrentChannels"=w329:i32[])
        n172 = for {
          tunnel: w333 -> [w341]
          shift-right: [w340] -> w332
          shift-left: errorcluster {"status"=FALSE, "code"=0, "source"=""} ("error out") -> [w339]
          tunnel: w329 -> [w335] mode=indexing
          tunnel: w328 -> [w338]
          n173 = Index Array(array=w338, index=w335) -> (element=w337:T2)
          n174 = Unbundle By Name(w337) -> ("Enable"=w336:bool)
          n175 = call "TH260_SetInputChannelEnable.vi"("error in (no error)"=w339, "enable"=w336, "channel"=w335, "devidx"=w341) -> ("error out"=w340:errorcluster)  [unwired: 6 in, 1 out]
        }
      }
      frame "SetInpChanOffset" {
        n176 = Unbundle By Name(w348) -> ("DevIdx"=w347:i32, "Channels"=w342:T2[], "CurrentChannels"=w343:i32[])
        n177 = for {
          tunnel: w347 -> [w353]
          shift-right: [w350] -> w346
          shift-left: errorcluster {"status"=FALSE, "code"=0, "source"=""} ("error out") -> [w351]
          tunnel: w343 -> [w352] mode=indexing
          tunnel: w342 -> [w355]
          n178 = Index Array(array=w355, index=w352) -> (element=w354:T2)
          n179 = Unbundle By Name(w354) -> ("Offset"=w349:i32)
          n180 = call "TH260_SetInputChannelOffset.vi"("error in (no error)"=w351, "offset"=w349, "channel"=w352, "devidx"=w353) -> ("error out"=w350:errorcluster)  [unwired: 6 in, 1 out]
        }
      }
      frame "SetInpChanCFD" {
        n181 = Unbundle By Name(w362) -> ("DevIdx"=w361:i32, "Channels"=w356:T2[], "CurrentChannels"=w357:i32[])
        n182 = for {
          tunnel: w361 -> [w365]
          shift-right: [w367] -> w360
          shift-left: errorcluster {"status"=FALSE, "code"=0, "source"=""} ("error out") -> [w368]
          tunnel: w357 -> [w366] mode=indexing
          tunnel: w356 -> [w370]
          n183 = Index Array(array=w370, index=w366) -> (element=w369:T2)
          n184 = Unbundle By Name(w369) -> ("CFDLevel"=w364:i32, "ZeroX"=w363:i32)
          n185 = call "TH260_SetInputCFD.vi"("channel"=w366, "error in (no error)"=w368, "CFD ZeroCross"=w363, "CFD Level"=w364, "devidx"=w365) -> ("error out"=w367:errorcluster)  [unwired: 5 in, 1 out]
        }
      }
      frame "SetInpChanTrg" {
        n186 = Unbundle By Name(w377) -> ("DevIdx"=w376:i32, "Channels"=w371:T2[], "CurrentChannels"=w372:i32[])
        n187 = for {
          tunnel: w376 -> [w380]
          shift-right: [w382] -> w375
          shift-left: errorcluster {"status"=FALSE, "code"=0, "source"=""} ("error out") -> [w383]
          tunnel: w372 -> [w381] mode=indexing
          tunnel: w371 -> [w385]
          n188 = Index Array(array=w385, index=w381) -> (element=w384:T2)
          n189 = Unbundle By Name(w384) -> ("TrgLevel"=w379:i32, "TrgEdge"=w378:i32)
          n190 = call "TH260_SetInputEdgeTrg.vi"("channel"=w381, "error in (no error)"=w383, "edge"=w378, "level"=w379, "devidx"=w380) -> ("error out"=w382:errorcluster)  [unwired: 5 in, 1 out]
        }
      }
      frame "SetInpChanDeadtime" {
        n191 = Unbundle By Name(w392) -> ("DevIdx"=w391:i32, "Channels"=w386:T2[], "CurrentChannels"=w387:i32[])
        n192 = for {
          tunnel: w391 -> [w394]
          shift-right: [w396] -> w390
          shift-left: errorcluster {"status"=FALSE, "code"=0, "source"=""} ("error out") -> [w397]
          tunnel: w387 -> [w395] mode=indexing
          tunnel: w386 -> [w399]
          n193 = Index Array(array=w399, index=w395) -> (element=w398:T2)
          n194 = Unbundle By Name(w398) -> ("dtcode"=w393:i32)
          n195 = call "TH260_SetInputDeadTime.vi"("error in (no error)"=w397, "dtcode"=w393, "channel"=w395, "devidx"=w394) -> ("error out"=w396:errorcluster)  [unwired: 6 in, 1 out]
        }
      }
      frame "SetSyncDivider" {
        n196 = Unbundle By Name(w407) -> ("DevIdx"=w406:i32, "SyncDivider"=w402:i32)
        n197 = Power Of 2(x=w402) -> (2^x=w401:dbl)
        n198 = To Long Integer(number=w401) -> (32bit integer=w400:i32)
        n199 = call "TH260_SetSyncDiv.vi"("SyncDivider"=w400, "devidx"=w406) -> ("error out"=w404:errorcluster)  [unwired: 8 in, 1 out]
        n200 = flat-sequence {
          tunnel: w404 -> [w408]
          tunnel: [w408] -> w403
          frame #0 {
            n201 = Wait (ms)(milliseconds to wait=u32 100) -> ()  [unwired: 1 out]
          }
        }
      }
      frame "SetSyncTrg" {
        n202 = Unbundle By Name(w415) -> ("DevIdx"=w412:i32, "SyncTrgLevel"=w410:i32, "SyncTrgEdge"=w411:i32)
        n203 = call "TH260_SetSyncEdgeTrg.vi"("edge"=w411, "level"=w410, "devidx"=w412) -> ("error out"=w413:errorcluster)  [unwired: 7 in, 1 out]
      }
      frame "SetSyncCFD" {
        n204 = Unbundle By Name(w421) -> ("DevIdx"=w418:i32, "SyncCFDLevel"=w416:i32, "SyncZeroX"=w417:i32)
        n205 = call "TH260_SetSyncCFD.vi"("CFD ZeroCross"=w417, "CFD Level"=w416, "devidx"=w418) -> ("error out"=w419:errorcluster)  [unwired: 7 in, 1 out]
      }
      frame "SetSyncOffset" {
        n206 = Unbundle By Name(w426) -> ("DevIdx"=w424:i32, "SyncOffset"=w423:i32)
        n207 = call "TH260_SetSyncChannelOffset.vi"("Offset"=w423, "devidx"=w424) -> ("error out"=w425:errorcluster)  [unwired: 8 in, 1 out]
      }
      frame "SetBinning" {
        # "When binning is changed the new resolution is querried"
        n208 = Unbundle By Name(w433) -> ("DevIdx"=w431:i32, "Binning"=w430:i32)
        n209 = call "TH260_SetBinning.vi"("Binning"=w430, "devidx"=w431) -> ("error out"=w432:errorcluster)  [unwired: 8 in, 1 out]
        n210 = Build Array (concatenate)(TH260_UIThread_Cmds."GetResolution", w428) -> (w429:T10[])
      }
      frame "SetHistoOffset" {
        n211 = Unbundle By Name(w438) -> ("DevIdx"=w435:i32, "HistoOffset"=w434:i32)
        n212 = call "TH260_SetOffset.vi"("Offset"=w434, "devidx"=w435) -> ("error out"=w436:errorcluster)  [unwired: 8 in, 1 out]
      }
      frame "SetStopOvl" {
        n213 = Unbundle By Name(w444) -> ("DevIdx"=w441:i32, "StopOvl."=w440:bool, "OvlLevel"=w439:u32)
        n214 = call "TH260_SetStopOverflow.vi"("stopcount"=w439, "StopOnOverflow"=w440, "devidx"=w441) -> ("error out"=w442:errorcluster)  [unwired: 7 in, 1 out]
      }
      frame "SetBitShift" {
        n215 = Unbundle By Name(w448) -> ("BitShift"=w446:i32, "SyncRate"=w447:i32)
        n216 = Negate(x=w446) -> (-x=w456:i32)
        n217 = Bundle By Name(cluster=T7 {"Cmd"=enum."Proc", "nActual"=0, "Buffer"=[], "TickCount"=0, "Param"=0} ("MH_DataProcThread_QData"), "Param"=w456, "Cmd"=TH260_DataProcThread_QCmds."SetShift") -> (w462:T7)
        n218 = To Double Precision Float(number=w446) -> (double precision float=w461:dbl)
        n219 = To Double Precision Float(number=w447) -> (double precision float=w460:dbl)
        n220 = Power Of 2(x=w461) -> (2^x=w459:dbl)
        n221 = Enqueue Element(queue=w449, element=w462) -> ()  [unwired: 2 in, 3 out]
        n222 = Multiply(x=w459, y=1000.0) -> (x*y=w458:dbl)
        n223 = Divide(x=w458, y=w460) -> (x/y=w445:dbl)
        "DeltaT" <- w445
        n224 = Bundle By Name(cluster=T5 {"Histos"=[], "Cmd"=enum."_none_", "TimeTrace"=[], "Bin"=0, "Total bin"=0, "Status"="", "Resol"=0.0, "DeltaT"=0.0, "nChannels"=0} ("MH_GUIThread_QData"), "DeltaT"=w445, "Cmd"=TH260_VisThread_QCmds."DeltaT") -> (w457:T5)
        n225 = Enqueue Element(queue=w450, element=w457) -> ()  [unwired: 2 in, 3 out]
      }
      frame "SetHistoAcqTime" {
        n226 = Unbundle By Name(w465) -> ("SyncRate"=w471:i32, "HistoAcqTime"=w464:dbl)
        n227 = To Double Precision Float(number=w471) -> (double precision float=w474:dbl)
        n228 = Multiply(x=w474, y=w464) -> (x*y=w473:dbl)
        n229 = Round To Nearest(number=w473) -> (nearest integer value=w472:dbl)
        n230 = To Long Integer(number=w472) -> (32bit integer=w470:i32)
        n231 = Bundle By Name(cluster=T7 {"Cmd"=enum."Proc", "nActual"=0, "Buffer"=[], "TickCount"=0, "Param"=0} ("MH_DataProcThread_QData"), "Param"=w470, "Cmd"=TH260_DataProcThread_QCmds."SetHistAcqTime") -> (w469:T7)
        n232 = Enqueue Element(queue=w466, element=w469) -> ()  [unwired: 2 in, 3 out]
      }
      frame "GetRates" {
        n233 = Unbundle By Name(w478) -> ("Init Info.nchannels"=w485:i32, "Channels"=w479:T2[], "DevIdx"=w480:i32)
        n234 = call "TH260_GetSyncRate.vi"("devidx"=w480) -> ("error out"=w484:errorcluster, "rate"=w476:i32)  [unwired: 8 in, 1 out]
        n235 = Format Into String(format string="Sync Rate: %d cps\n", w476) -> (resulting string=→"SyncRate":string)  [unwired: 2 in, 1 out]
        n236 = for {
          N: w485 -> [_]
          tunnel: w480 -> [w493]
          tunnel: [w490] -> w482 mode=indexing
          shift-right: [w492] -> w486
          shift-left: w484 -> [w494]
          tunnel: w479 -> [w489] mode=indexing
          i -> [w491]
          n237 = Unbundle By Name(w489) -> ("Enable"=w488:bool)
          n238 = case shown="True" w488 {
            tunnel: w494 -> [w495 w500]
            tunnel: w493 -> [_ w499]
            tunnel: [w495 w498] -> w492
            tunnel: w491 -> [_ w497]
            tunnel: [_ w496] -> w490
            frame False {
            }
            frame True {
              n239 = call "TH260_GetCountRate.vi"("error in (no error)"=w500, "Channel"=w497, "devidx"=w499) -> ("error out"=w498:errorcluster, "rate"=w496:i32)  [unwired: 6 in, 1 out]
            }
          }
        }
        "CountRates" <- w482
        n240 = Bundle By Name(cluster=w478, "SyncRate"=w476) -> (w477:T8)
      }
      frame "StartMeas" {
        n241 = Bundle By Name(cluster=T7 {"Cmd"=enum."Proc", "nActual"=0, "Buffer"=[], "TickCount"=0, "Param"=0} ("MH_DataProcThread_QData"), "Cmd"=TH260_DataProcThread_QCmds."Init") -> (w502:T7)
        n242 = Unbundle By Name(w511) -> ("DevIdx"=w509:i32, "AcqTime"=w505:i32)
        n243 = Enqueue Element(queue=w504, element=w502) -> ()  [unwired: 2 in, 3 out]
        n244 = call "TH260_StartMeas.vi"("Acquisition time"=w505, "devidx"=w509) -> ("error out"=w510:errorcluster)  [unwired: 8 in, 1 out]
        n245 = Build Array (concatenate)(w508, TH260_UIThread_Cmds."ReadFiFo") -> (w507:T10[])
      }
      frame "StopMeas" {
        n246 = Unbundle By Name(w517) -> ("Run cont."=w512:bool, "DevIdx"=w518:i32)
        n247 = call "TH260_StopMeas.vi"("devidx"=w518) -> ("error out"=w519:errorcluster)  [unwired: 9 in, 1 out]
        n248 = case shown="True" w512 {
          tunnel: w517 -> [w523 w525]
          tunnel: [w522 w525] -> w516
          tunnel: [w520 w524] -> w515
          frame False {
            w520 = T10[] [enum."ReadFiFo"] items=["Idle", "Init", "SetInpChanEnable", "SetInpChanOffset", "SetInpChanCFD", "SetInpChanTrg", "SetInpChanDeadtime", "SetSyncDivider", "SetSyncCFD", "SetSyncTrg", "SetSyncOffset", "SetBinning", "SetHistoOffset", "SetHistoLen", "SetStopOvl", "SetBitShift", "SetHistoAcqTime", "GetRates", "StartMeas", "StopMeas", "AbortMeas", "GetResolution", "GetHisto", "ReadFiFo", "WriteStatus", "Resize", "EnableControls", "DisableControls", "Error", "Exit"]
            w521 = FALSE ("StartMeas")
            n249 = Bundle By Name(cluster=w523, "StartMeas"=w521) -> (w522:T8)
            n250 = local write "Start"(w521) -> ()
          }
          frame True {
            w524 = T10[] [enum."ReadFiFo", enum."StartMeas"] items=["Idle", "Init", "SetInpChanEnable", "SetInpChanOffset", "SetInpChanCFD", "SetInpChanTrg", "SetInpChanDeadtime", "SetSyncDivider", "SetSyncCFD", "SetSyncTrg", "SetSyncOffset", "SetBinning", "SetHistoOffset", "SetHistoLen", "SetStopOvl", "SetBitShift", "SetHistoAcqTime", "GetRates", "StartMeas", "StopMeas", "AbortMeas", "GetResolution", "GetHisto", "ReadFiFo", "WriteStatus", "Resize", "EnableControls", "DisableControls", "Error", "Exit"]
          }
        }
        n251 = Build Array (concatenate)(w514, w515) -> (w513:T10[])
      }
      frame "AbortMeas" {
        w527 = FALSE ("StartMeas")
        n252 = Unbundle By Name(w529) -> ("DevIdx"=w530:i32)
        n253 = call "TH260_StopMeas.vi"("devidx"=w530) -> ("error out"=w531:errorcluster)  [unwired: 9 in, 1 out]
        n254 = Bundle By Name(cluster=w529, "StartMeas"=w527) -> (w528:T8)
        n255 = local write "Start"(w527) -> ()
      }
      frame "GetResolution" {
        # "Resolution in ns"
        # "Gets resolution in ps"
        # "Resolution is saved in UIThread Data cluster in ns"
        n256 = Unbundle By Name(w540) -> ("DevIdx"=w542:i32)
        n257 = call "TH260_GetResolution.vi"("devidx"=w542) -> ("error out"=w541:errorcluster, "resolution"=w538:dbl)  [unwired: 8 in, 1 out]
        n258 = Divide(x=w538, y=1000.0) -> (x/y=w534:dbl)
        n259 = Bundle By Name(cluster=w540, "Resolution"=w534) -> (w539:T8)
        n260 = Bundle By Name(cluster=T5 {"Histos"=[], "Cmd"=enum."_none_", "TimeTrace"=[], "Bin"=0, "Total bin"=0, "Status"="", "Resol"=0.0, "DeltaT"=0.0, "nChannels"=0} ("MH_GUIThread_QData"), "Resol"=w534, "Cmd"=TH260_VisThread_QCmds."Resol") -> (w532:T5)
        n261 = Enqueue Element(queue=w536, element=w532) -> ()  [unwired: 2 in, 3 out]
      }
      frame "ReadFiFo" {
        w552 = 2  # FLAG_FIFOFULL
        # "Reads photon records from HW and transferes them to DataProcThread via Queue."
        n262 = Unbundle By Name(w554) -> ("DevIdx"=w548:i32)
        n263 = call "TH260_GetFlags.vi"("devidx"=w548) -> ("error out"=w550:errorcluster, "flags"=w551:i32)  [unwired: 8 in, 1 out]
        n264 = And(x=w551, y=w552) -> (x .and. y?=w553:i32)
        n265 = Not Equal To 0?(x=w553) -> (x != 0?=w547:bool)
        "OverRun" <- w547
        n266 = case shown="False" w547 {
          tunnel: w550 -> [w564 w567]
          tunnel: [w563 w567] -> w549
          tunnel: w548 -> [w556 _]
          tunnel: w546 -> [w562 _]
          tunnel: w545 -> [w561 _]
          tunnel: [w561 w565] -> w544
          frame False {
            n267 = call "TH260_ReadFiFo.vi"("error in (no error)"=w564, "devidx"=w556) -> ("error out"=w563:errorcluster, "nactual"=w555:i32, "buffer"=w559:u32[])  [unwired: 6 in, 1 out]
            n268 = Bundle By Name(cluster=T7 {"Cmd"=enum."Proc", "nActual"=0, "Buffer"=[], "TickCount"=0, "Param"=0} ("MH_DataProcThread_QData"), "Buffer"=w559, "nActual"=w555, "Cmd"=TH260_DataProcThread_QCmds."Proc") -> (w557:T7)
            n269 = Enqueue Element(queue=w562, element=w557) -> ()  [unwired: 2 in, 3 out]
          }
          frame True {
            n270 = Build Array(TH260_UIThread_Cmds."AbortMeas") -> (w565:T10[])
          }
        }
      }
      frame "WriteStatus" {
        n271 = Unbundle By Name(w569) -> ("Status"=→"Status":string)
      }
      frame "Resize" {
        n272 = property on="Pane 3" class="Pane"() -> ("Width"=w576:u32)  [unwired: 2 in, 2 out]
        n273 = Subtract(x=w576, y=i16 100 ("b")) -> (x-y=w582:u32)
        n274 = Unbundle By Name(w571) -> ("Init Info.nchannels"=w579:i32)
        n275 = Quotient & Remainder(x=w582, y=i16 99 ("m")) -> (floor(x/y)=w581:u32)  [unwired: 1 out]
        n276 = In Range and Coerce(upper limit=w579, x=w581, lower limit=4) -> (coerced(x)=w580:u32)  [unwired: 1 out]
        n277 = Equal?(x=w579, y=w580) -> (x = y?=w578:bool)
        n278 = Not(x=w578) -> (.not. x?=w577:bool)
        n279 = property on="Channels" class="Arr (strict)"("HorizScroll"=w577, "Number of Columns"=w580, "Index Values"=u32[] [0]) -> ()  [unwired: 2 in, 2 out]
      }
      frame "EnableControls" {
        n280 = property class="VI"() -> ("Panel"=w587:refnum<vi>)  [unwired: 2 in, 2 out]
        n281 = property class="Pnl"(reference=w587) -> ("Controls[]"=w586:refnum<vi>[])  [unwired: 1 in, 2 out]
        n282 = property class="Pnl"(reference=w587) -> ("Decos[]"=w588:refnum<vi>[])  [unwired: 1 in, 2 out]
        n283 = for {
          tunnel: w588 -> [w592] mode=indexing
          tunnel: TRUE -> [w591]
          n284 = property class="Decor"(reference=w592, "Visible"=w591) -> ()  [unwired: 1 in, 2 out]
        }
        n285 = for {
          tunnel: w586 -> [w595] mode=indexing
          tunnel: T11."Enabled" ("Disabled") -> [w594]
          tunnel: [w593] -> _
          n286 = property class="Ctl"(reference=w595, "DisabledEnum"=w594) -> (error out=w593:errorcluster)  [unwired: 1 in, 1 out]
        }
      }
      frame "DisableControls" {
        n287 = property class="VI"() -> ("Panel"=w599:refnum<vi>)  [unwired: 2 in, 2 out]
        n288 = property class="Pnl"(reference=w599) -> ("Controls[]"=w598:refnum<vi>[])  [unwired: 1 in, 2 out]
        n289 = property class="Pnl"(reference=w599) -> ("Decos[]"=w600:refnum<vi>[])  [unwired: 1 in, 2 out]
        n290 = for {
          tunnel: w600 -> [w604] mode=indexing
          tunnel: FALSE -> [w603]
          n291 = property class="Decor"(reference=w604, "Visible"=w603) -> ()  [unwired: 1 in, 2 out]
        }
        n292 = for {
          tunnel: w598 -> [w607] mode=indexing
          tunnel: T11."Disabled and Grayed Out" ("Disabled") -> [w606]
          tunnel: [w605] -> _
          n293 = property class="Ctl"(reference=w607, "DisabledEnum"=w606) -> (error out=w605:errorcluster)  [unwired: 1 in, 1 out]
        }
      }
      frame "Error" {
        w608 = T10[] [enum."Exit"] items=["Idle", "Init", "SetInpChanEnable", "SetInpChanOffset", "SetInpChanCFD", "SetInpChanTrg", "SetInpChanDeadtime", "SetSyncDivider", "SetSyncCFD", "SetSyncTrg", "SetSyncOffset", "SetBinning", "SetHistoOffset", "SetHistoLen", "SetStopOvl", "SetBitShift", "SetHistoAcqTime", "GetRates", "StartMeas", "StopMeas", "AbortMeas", "GetResolution", "GetHisto", "ReadFiFo", "WriteStatus", "Resize", "EnableControls", "DisableControls", "Error", "Exit"]
        w611 = T14 1 items=["no dialog", "OK message", "continue or stop message", "OK message + warnings", "continue/stop + warnings"] ("type of dialog (OK msg:1)")
        # "Error case: If an error occures the user is informed and the programm terminates. Add your own code to handle error events (e.g. exception lists, etc.)"
        n294 = call <vilib>:"Simple Error Handler.vi"("type of dialog (OK msg:1)"=w611, "error in (no error)"=w610) -> ()  [unwired: 3 in, 5 out]
      }
      frame "Exit" {
        n295 = Release Queue(queue=w613) -> ()  [unwired: 2 in, 3 out]
        n296 = Release Queue(queue=w612) -> ()  [unwired: 2 in, 3 out]
        n297 = Unbundle By Name(w617) -> ("DevIdx"=w616:i32)
        n298 = call "TH260_CloseDevice.vi"("devidx"=w616) -> ("error out"=w615:errorcluster)  [unwired: 9 in, 1 out]
      }
    }
    n299 = call "TH260_EnQError.vi"("error in (no error)"=w24, "Cmds_in"=w22) -> ("error out"=w23:errorcluster, "Cmds_out"=w21:T10[])  [unwired: 8 in]
  }
  n300 = call "TH260_DataProcThread.vi"("TH260_VisThread_QRef"=w7, "TH260_DataProcThread_QRef"=w1) -> ()  [unwired: 10 in]
  n301 = while {
    tunnel: w7 -> [w626]
    shift-right: [w622] -> _
    shift-left: T4 {"Resol"=0.0, "DeltaT"=0.0, "NumChannels"=0} -> [w623]
    tunnel: w1 -> [w621]
    stop <- w619 stop-if-true
    # "VisualizationThread"
    n302 = Dequeue Element(queue=w626, timeout in ms (-1)=100) -> (element=w624:T5, error out=w619:errorcluster)  [unwired: 1 in, 2 out]
    n303 = Unbundle By Name(w624) -> ("Cmd"=w625:T6)
    n304 = case shown="\"Histo\"" w625 {
      tunnel: w624 -> [_ w639 w641 w653 w661 w665 w669]
      tunnel: w623 -> [w629 w637 w643 w645 w660 w664 w668]
      tunnel: [w629 w637 w642 w645 w660 w663 w667] -> w622
      tunnel: w621 -> [w628 _ _ _ w657 _ _]
      tunnel: w619 -> [w627 _ _ _ _ _ _]
      frame "_none_", Default {
        n305 = case shown="No Error" w627 {
          tunnel: w628 -> [w633 _]
          frame No Error {
            n306 = Get Queue Status(queue=w633) -> (# elements in queue=w631:i32)  [unwired: 2 in, 7 out]
            n307 = Format Into String(format string="Elements in Q: %d", w631) -> (resulting string=w630:string)  [unwired: 2 in, 1 out]
            n308 = local write "Status"(w630) -> ()
          }
          frame Error {
          }
        }
      }
      frame "Histo" {
        n309 = Unbundle By Name(w639) -> ("Histos"=w634:u32[][])
        n310 = Unbundle By Name(w637) -> ("Resol"=w636:dbl)
        n311 = Bundle(0.0, "Resol"=w636, "Histos"=w634) -> (→"HistoGraph":cluster{dbl, "Resol":dbl, "Histos":u32[][]})  [unwired: 1 in]
      }
      frame "nChannels" {
        n312 = Unbundle By Name(w641) -> ("nChannels"=w640:i32)
        n313 = Bundle By Name(cluster=w643, "NumChannels"=w640) -> (w642:T4)
      }
      frame "TTrace" {
        n314 = Unbundle By Name(w653) -> ("Total bin"=w652:u64, "Bin"=w651:i32, "TimeTrace"=w650:u32[][])
        n315 = Unbundle By Name(w645) -> ("DeltaT"=w644:dbl)
        n316 = call "TH260_TTraceToGraph.vi"("DeltaT"=w644, "TimeTrace"=w650, "Bin"=w651, "Total bin"=w652) -> ("TimeTrace_out"=w647:u32[][], "dt"=w648:dbl, "T0"=w649:dbl)  [unwired: 5 in]
        n317 = Bundle("T0"=w649, "dt"=w648, "TimeTrace_out"=w647) -> (→"TTraceGraph":T15)  [unwired: 1 in]
      }
      frame "Status" {
        n318 = Unbundle By Name(w661) -> ("Status"=w658:string)
        n319 = Get Queue Status(queue=w657) -> (# elements in queue=w656:i32)  [unwired: 2 in, 7 out]
        n320 = Format Into String(format string="\t\tElements in Q: %d", w656) -> (resulting string=w654:string)  [unwired: 2 in, 1 out]
        n321 = Concatenate Strings(w658, w654) -> (w659:string)
        n322 = local write "Status"(w659) -> ()
      }
      frame "DeltaT" {
        n323 = Unbundle By Name(w665) -> ("DeltaT"=w662:dbl)
        n324 = Bundle By Name(cluster=w664, "DeltaT"=w662) -> (w663:T4)
      }
      frame "Resol" {
        n325 = Unbundle By Name(w669) -> ("Resol"=w666:dbl)
        n326 = Bundle By Name(cluster=w668, "Resol"=w666) -> (w667:T4)
      }
    }
  }
